vi "Write Value.vi"(8 "error in (no error)":errorcluster, 10 "Value":u32, 11 "Block in":refnum<class "Block.lvclass">) -> (0 "error out":errorcluster, 3 "Block out":refnum<class "Block.lvclass">)   [LabVIEW 2017, in "Block.lvclass"]
uses:
  Block.lvclass
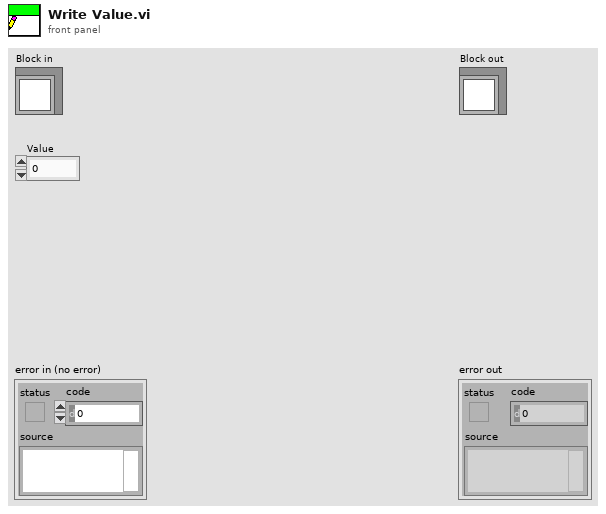
[diagram p1: front panel]
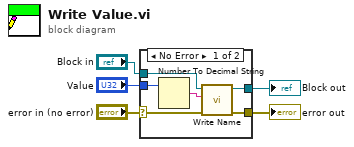
[diagram p0: block diagram]
diagram:
  n1 = case shown="No Error" "error in (no error)" {
    selector: "error in (no error)" -> [w6 w12]
    tunnel: [w8 w12] -> w4
    tunnel: [w9 w13] -> w2
    tunnel: "Block in" -> [w10 w13]
    tunnel: "Value" -> [w11 _]
    frame No Error {
      n2 = Number To Decimal String(number=w11) -> (decimal integer string=w7:string)  [unwired: 1 in]
      n3 = call-dynamic "Write Name.vi"("error in (no error)"=w6, "Name"=w7, "Block in"=w10) -> ("error out"=w8:errorcluster, "Block out"=w9:refnum<class "Block.lvclass">)  [unwired: 7 in]
    }
    frame Error {
    }
  }
  "error out" <- w4
  "Block out" <- w2
